vi "Solve General Linear Equations with SVD (DBL, multi hand).vi"(8 "iteration":i32=2, 9 "relative tolerance":dbl, 10 "Known Matrix":T1, 11 "Input Matrix":T1) -> (0 "error":i32, 3 "Solution Matrix":T1)   [LabVIEW 2018, in "NI_AALPro.lvlib"]
uses:
  NI_AALPro.lvlib
  RealMatrix.ctl
  Real Transpose Matrix.vi
  A x Vector.vi
  Real SVD Decomposition.vi
  NI_AALBase.lvlib
  NI_Matrix.lvlib
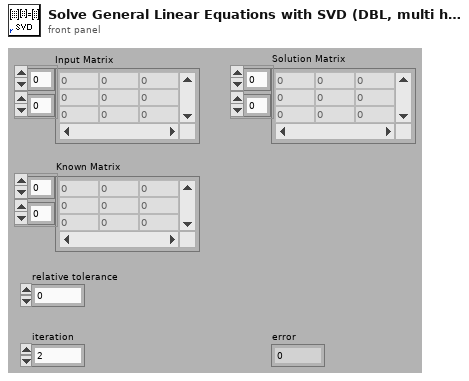
[diagram p1: front panel]
types:
  T1 = typedef "NI_Matrix.lvlib/RealMatrix.ctl" = dbl[][]
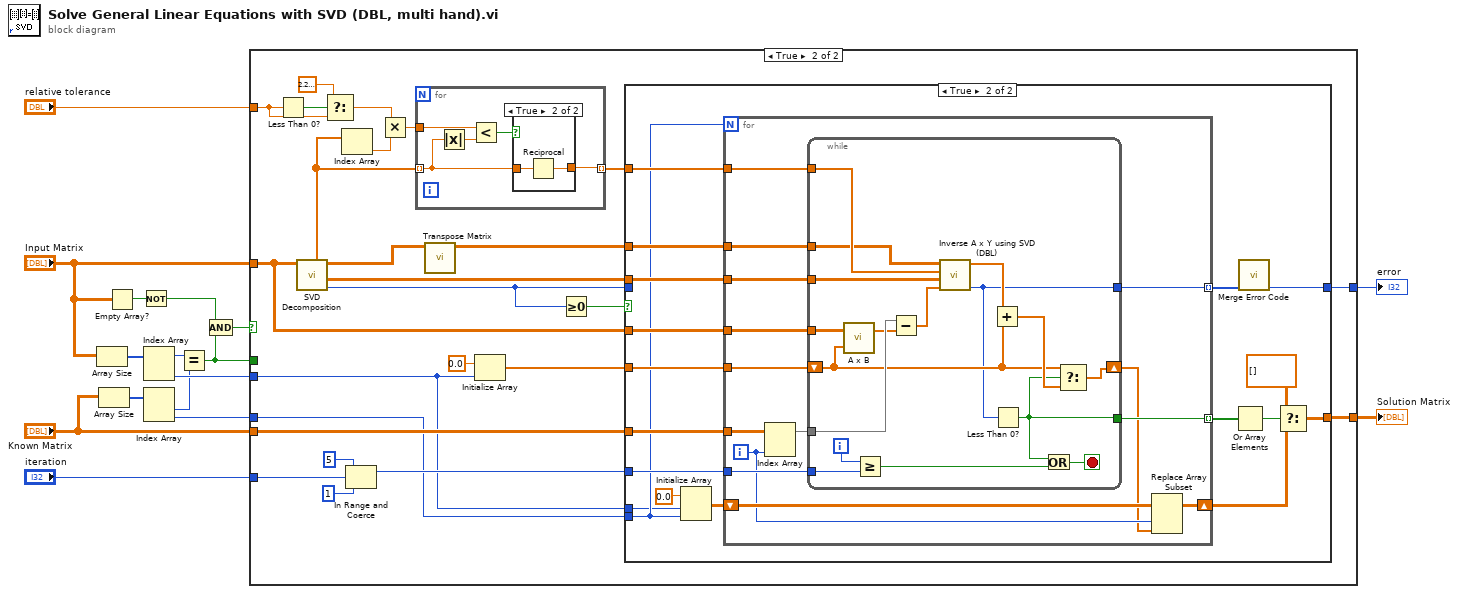
[diagram p0: block diagram]
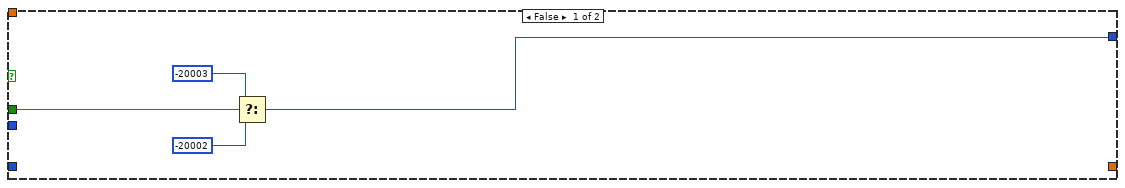
[diagram p2: hidden frame]
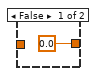
[diagram p4: hidden frame]
diagram:
  n1 = Array Size(array="Input Matrix") -> (size(s)=w14:i32[])
  n2 = Array Size(array="Known Matrix") -> (size(s)=w9:i32[])
  n3 = Empty Array?(array="Input Matrix") -> (empty?=w5:bool)
  n4 = Not(x=w5) -> (.not. x?=w4:bool)
  n5 = Index Array(array=w14) -> (element #1=w8:i32, element #2=w11:i32)  [unwired: 2 in]
  n6 = Index Array(array=w9) -> (element #1=w7:i32, element #2=w1:i32)  [unwired: 2 in]
  n7 = Equal?(x=w8, y=w7) -> (x = y?=w2:bool)
  n8 = Compound Arithmetic op=AND(w4, w2) -> (w3:bool)
  n9 = case shown="True" w3 {
    tunnel: "relative tolerance" -> [_ w44]
    tunnel: "iteration" -> [_ w34]
    tunnel: "Input Matrix" -> [_ w23]
    tunnel: w11 -> [_ w21]
    tunnel: [w17 w27] -> w13
    tunnel: "Known Matrix" -> [_ w25]
    tunnel: [_ w24] -> w12
    tunnel: w2 -> [w20 _]
    tunnel: w1 -> [_ w22]
    frame False {
      n10 = Select(t=-20003, s=w20, f=-20002) -> (s? t:f=w17:i32)
    }
    frame True {
      n11 = Less Than 0?(x=w44) -> (x < 0?=w45:bool)
      n12 = call-poly "SVD Decomposition.vi"("A"=w23) -> ("error"=w26:i32, "Matrix V"=w37:T1, "Matrix U"=w38:T1, "Vector S"=w39:dbl[])  [unwired: 6 in, 1 out]
      n13 = Select(t=2.220446049250313e-16, s=w45, f=w44) -> (s? t:f=w42:dbl)
      n14 = Index Array(array=w39) -> (element=w41:dbl)  [unwired: 1 in]
      n15 = In Range and Coerce(upper limit=5, x=w34, lower limit=1) -> (coerced(x)=w31:i32)  [unwired: 1 out]
      n16 = Multiply(x=w42, y=w41) -> (x*y=w40:dbl)
      n17 = for {
        tunnel: w39 -> [w98] mode=indexing
        tunnel: w40 -> [w100]
        tunnel: [w96] -> w30 mode=indexing
        n18 = Absolute Value(x=w98) -> (abs(x)=w99:dbl)
        n19 = Less?(x=w100, y=w99) -> (x < y?=w97:bool)
        n20 = case shown="True" w97 {
          tunnel: w98 -> [_ w103]
          tunnel: [0.0 w102] -> w96
          frame False {
          }
          frame True {
            n21 = Reciprocal(x=w103) -> (1/x=w102:dbl)
          }
        }
      }
      n22 = call-poly "Transpose Matrix.vi"("Input Matrix"=w38) -> ("Matrix Transpose"=w36:T1)  [unwired: 9 in, 1 out]
      n23 = Initialize Array(0.0 ("element"), w21) -> (w28:dbl[])
      n24 = Greater Or Equal To 0?(x=w26) -> (x >= 0?=w35:bool)
      n25 = case shown="True" w35 {
        tunnel: w37 -> [_ w61]
        tunnel: w36 -> [_ w62]
        tunnel: w23 -> [_ w59]
        tunnel: w25 -> [_ w60]
        tunnel: w31 -> [_ w64]
        tunnel: w30 -> [_ w63]
        tunnel: w28 -> [_ w58]
        tunnel: [_ w55] -> w24
        tunnel: [w46 w52] -> w27
        tunnel: w26 -> [w46 _]
        tunnel: w22 -> [_ w51]
        tunnel: w21 -> [_ w49]
        frame False {
        }
        frame True {
          n26 = Initialize Array(0.0 ("element"), w49, w51) -> (w48:dbl[][])
          n27 = for {
            N: w51 -> [_]
            tunnel: w64 -> [w78]
            tunnel: w63 -> [w77]
            tunnel: w62 -> [w76]
            tunnel: w61 -> [w75]
            tunnel: w60 -> [w70]
            tunnel: w59 -> [w74]
            tunnel: w58 -> [w73]
            tunnel: [w72] -> w53 mode=indexing
            tunnel: [w69] -> w57 mode=indexing
            shift-right: [w66] -> w47
            shift-left: w48 -> [w68]
            i -> [w67]
            n28 = Index Array(array=w70, index (col)=w67) -> (element=w71:dbl[])  [unwired: 1 in]
            n29 = while {
              tunnel: w78 -> [w87]
              tunnel: w77 -> [w95]
              tunnel: w76 -> [w94]
              tunnel: w75 -> [w93]
              tunnel: w71 -> [w91]
              tunnel: w74 -> [w92]
              shift-right: [w82] -> w65
              shift-left: w73 -> [w81]
              tunnel: [w80] -> w72
              tunnel: [w79] -> w69
              i -> [w88]
              stop <- w85 stop-if-true
              n30 = call-poly "A x B.vi"("Vector"=w81, "A"=w92) -> ("A x Vector"=w90:dbl[])  [unwired: 1 out]
              n31 = Greater Or Equal?(x=w88, y=w87) -> (x >= y?=w86:bool)
              n32 = Subtract(x=w91, y=w90) -> (x-y=w89:dbl[])
              n33 = call "Inverse A x Y using SVD (DBL).vi"("Known Vector"=w89, "V"=w93, "1/S"=w95, "U*"=w94) -> ("error"=w80:i32, "Solution Vector"=w84:dbl[])  [unwired: 6 in]
              n34 = Add(x=w84, y=w81) -> (x+y=w83:dbl[])
              n35 = Less Than 0?(x=w80) -> (x < 0?=w79:bool)
              n36 = Or(x=w79, y=w86) -> (x .or. y?=w85:bool)
              n37 = Select(t=w81, s=w79, f=w83) -> (s? t:f=w82:dbl[])
            }
            n38 = Replace Array Subset(array=w68, new element=w65, index (col)=w67) -> (w66:dbl[][])  [unwired: 1 in]
          }
          n39 = Or Array Elements(Boolean array=w57) -> (logical OR=w56:bool)
          n40 = call "Merge Error Code.vi"("Error Code"=w53) -> ("error code"=w52:i32)  [unwired: 10 in]
          n41 = Select(t=dbl[][] [], s=w56, f=w47) -> (s? t:f=w55:dbl[][])
        }
      }
    }
  }
  "error" <- w13
  "Solution Matrix" <- w12
